vi "Translate_TEXT.vi"(8 "error In":errorcluster, 10 "Cle":string, 11 "Txt Refnum":refnum<vi>) -> (0 "error out":errorcluster)   [LabVIEW 2011]
uses:
  Dictionnary/EnumCommandDictionnaire.ctl
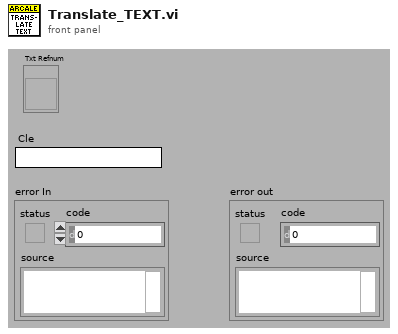
[diagram p1: front panel]
types:
  T1 = typedef "EnumCommandDictionnaire.ctl" = enum16{"Load", "Translate", "Save", "GetDico", "Set : A traduire = Vrai", "Set : A Traduire = Faux", "SetDico"}
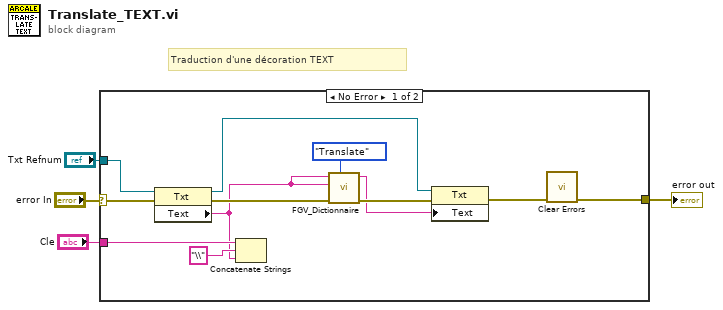
[diagram p0: block diagram]
diagram:
  # "Traduction d'une décoration TEXT"
  n1 = case shown="No Error" "error In" {
    selector: "error In" -> [w11 w17]
    tunnel: [w6 w17] -> w4
    tunnel: "Txt Refnum" -> [w13 _]
    tunnel: "Cle" -> [w12 _]
    frame No Error {
      n2 = property class="Txt"(reference=w13, error in=w11) -> (reference out=w15:refnum<vi>, error out=w9:errorcluster, "Text"=w5:string)
      n3 = Concatenate Strings(w12, "\\" ("string"), w5) -> ()  [unwired: 1 out]
      n4 = call "FGV_Dictionnaire.vi"("Command"=EnumCommandDictionnaire."Translate", "error in (no error)"=w9, "Chaîne"=w5, "Clé"=w5) -> ("error out"=w8:errorcluster, "Traduction"=w7:string)  [unwired: 5 in, 1 out]
      n5 = property class="Txt"(reference=w15, error in=w8, "Text"=w7) -> (error out=w14:errorcluster)  [unwired: 1 out]
      n6 = call <vilib>:"Clear Errors.vi"("error in (no error)"=w14) -> ("error out"=w6:errorcluster)  [unwired: 6 in]
    }
    frame Error {
    }
  }
  "error out" <- w4
